vi "Init Task.vi"(6 "line grouping":i32(ring) items=["one channel for each line", "one channel for all lines"], 7 "counter":tag, 8 "error in (no error)":errorcluster, 9 "name":string, 10 "physical channels":tag, 11 "DAQmxTaskCounterDigital in":refnum<class "DAQmxTaskCounterDigital.lvclass">) -> (0 "error out":errorcluster, 3 "DAQmxTaskCounterDigital out":refnum<class "DAQmxTaskCounterDigital.lvclass">)   [LabVIEW 2015, in "DAQmxTaskCounterDigital.lvclass"]
uses:
  DAQmxTaskCounterDigital.lvclass
  DAQmxTask.lvclass/DAQmxTask.ctl
  <vilib>/DAQmx/create/channels.llb/DAQmx Create Channel (CI-Count Edges).vi
  DAQmxTask.lvclass
  <resource>/objmgr/daqmx.rc
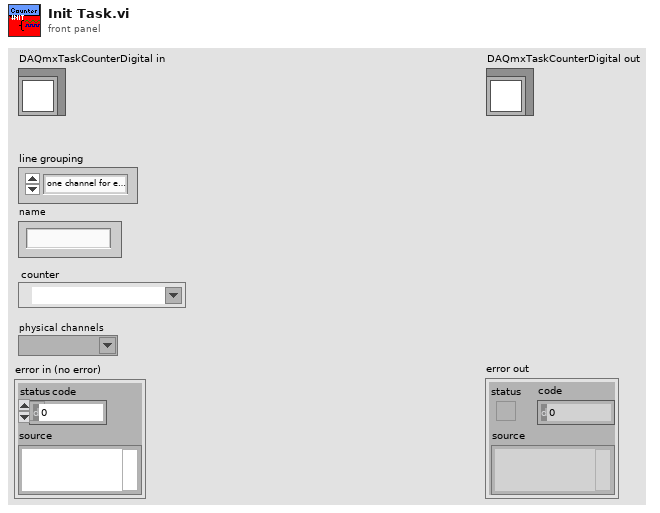
[diagram p1: front panel]
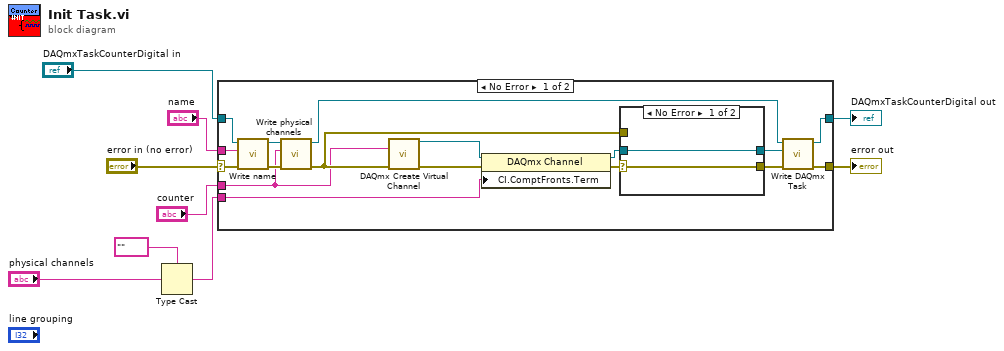
[diagram p0: block diagram]
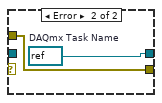
[diagram p2: hidden frame]
diagram:
  n1 = Type Cast(type=tag "" ("CI.ComptFronts.Term"), x="physical channels") -> (*(type *) &x=w2:tag)
  n2 = case shown="No Error" "error in (no error)" {
    selector: "error in (no error)" -> [w26 w32]
    tunnel: [w21 w32] -> w5
    tunnel: [w22 w31] -> w8
    tunnel: "name" -> [w18 _]
    tunnel: "DAQmxTaskCounterDigital in" -> [w17 w31]
    tunnel: "counter" -> [w12 _]
    tunnel: w2 -> [w10 _]
    frame No Error {
      n3 = call "Write name.vi"("error in (no error)"=w26, "name"=w18, "DAQmxTask in"=w17) -> ("error out"=w24:errorcluster, "DAQmxTask out"=w25:refnum<class "DAQmxTaskCounterDigital.lvclass">)  [unwired: 7 in]
      n4 = call "Write physical channels.vi"("error in (no error)"=w24, "physical channels"=w12, "DAQmxTask in"=w25) -> ("error out"=w15:errorcluster, "DAQmxTask out"=w23:refnum<class "DAQmxTaskCounterDigital.lvclass">)  [unwired: 7 in]
      n5 = call-poly <vilib>:"DAQmx Create Virtual Channel.vi"("counter"=w12, "error in"=w15) -> ("task out"=w13:refnum<k21>, "error out"=w16:errorcluster)  [unwired: 12 in]
      n6 = property class="DAQmx Channel"(reference=w13, error in=w16, "CI.ComptFronts.Term"=w10) -> (reference out=w14:refnum<k21>, error out=w11:errorcluster)
      n7 = case shown="No Error" w11 {
        selector: w11 -> [w28 _]
        tunnel: [w27 w29] -> w19
        tunnel: [w28 w30] -> w20
        tunnel: w15 -> [_ w30]
        tunnel: w14 -> [w27 _]
        frame No Error {
        }
        frame Error {
          w29 = refnum<k21> refnum  # DAQmx Task Name
        }
      }
      n8 = call "Write DAQmx Task.vi"("error in (no error)"=w20, "DAQmx Task Name"=w19, "DAQmxTask in"=w23) -> ("error out"=w21:errorcluster, "DAQmxTask out"=w22:refnum<class "DAQmxTaskCounterDigital.lvclass">)  [unwired: 7 in]
    }
    frame Error {
    }
  }
  "error out" <- w5
  "DAQmxTaskCounterDigital out" <- w8
